vi "Mapping Simulated Spectrum v10.0.0.vi"() -> (0 "Simulated Spectrum":cluster{i32[], dbl[]})   [LabVIEW 2010]
panel:
  out "Y (2D)":dbl[](array[numeric])
  out "X (1D)":i32[](array[numeric])
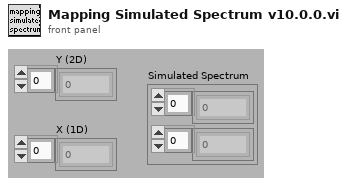
[diagram p1: front panel]
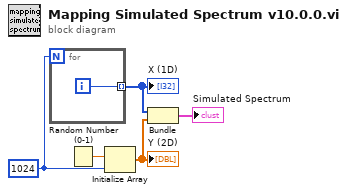
[diagram p0: block diagram]
diagram:
  w5 = 1024 ("Dimension")
  n1 = for {
    N: w5 -> [_]
    tunnel: [w6] -> w3 mode=indexing
    i -> [w6]
  }
  "X (1D)" <- w3
  n2 = Random Number (0-1)() -> (number: 0 to 1=w4:dbl)
  n3 = Initialize Array(w4, w5) -> (w2:dbl[])
  "Y (2D)" <- w2
  n4 = Bundle(w3, w2) -> (→"Simulated Spectrum":cluster{i32[], dbl[]})  [unwired: 1 in]
